vi "UnitTest-TimeLimitReliabilitycheck.vi"(8 "error in (no error)":errorcluster) -> (0 "error out":errorcluster)   [LabVIEW 2014]
uses:
  TableLogger_Actor/TableLoggerConfig.ctl
  TableLogger_Actor/TableLoggerTypes.ctl
  TableLogger_Actor/TableLoggerBackupConfig.ctl
  <vilib>/addons/_JKI Toolkits/Caraya/classes/Test/Test.lvclass
  TableLogger_Actor/TableLogger_Actor.lvlib
  <vilib>/addons/_JKI Toolkits/Caraya/classes/Assert/Assert.lvclass
panel:
  # "Connector Pane"
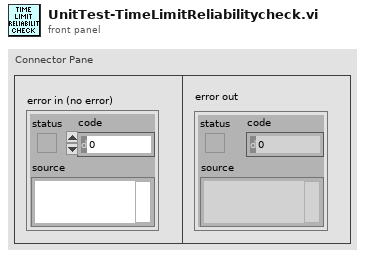
[diagram p1: front panel]
types:
  T1 = typedef "TableLogger_Actor.lvlib/TableLoggerConfig.ctl" = cluster{"TableLogger":T2, "DB File Path":path, "DB Backup Config":T3}
  T2 = typedef "TableLogger_Actor.lvlib/TableLoggerTypes.ctl" = enum16{"CSV Logger", "SQLite Logger"}
  T3 = typedef "TableLogger_Actor.lvlib/TableLoggerBackupConfig.ctl" = cluster{"Directory":path, "UTC Time Format":bool, "On Launch":bool, "Interval (Hours)":dbl, "Size Multiples (Bytes)":i32}
  T4 = typedef "TableLogger_Actor.lvlib/TableLoggerDataCluster.ctl" = cluster{"Numeric Data":i32, "Float Data":dbl, "String Data":string, "Enum Data":enum16{"Enum Item 1", "Enum Item 2"}, "Array Data":i32[]}
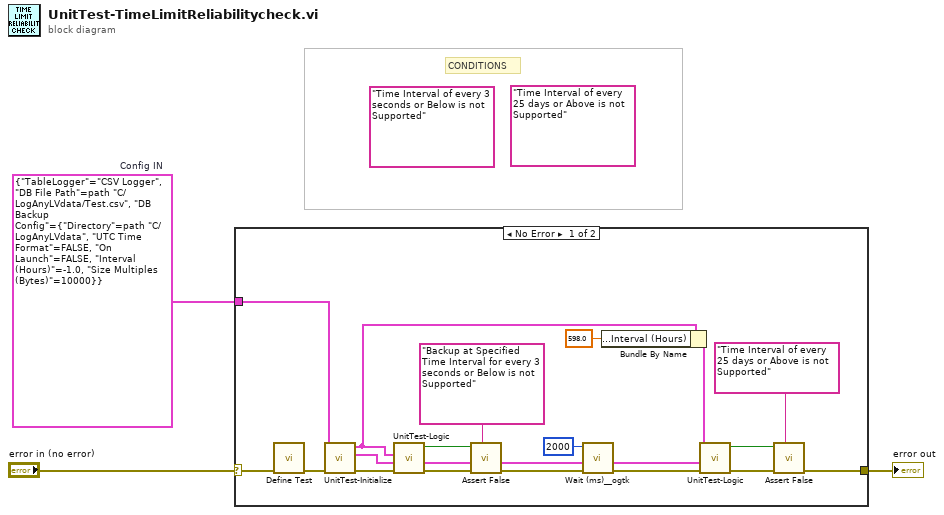
[diagram p0: block diagram]
diagram:
  w3 = T1 {"TableLogger"=enum."CSV Logger", "DB File Path"=path "C:/LogAnyLVdata/Test.csv", "DB Backup Config"={"Directory"=path "C:/LogAnyLVdata", "UTC Time Format"=FALSE, "On Launch"=FALSE, "Interval (Hours)"=-1.0, "Size Multiples (Bytes)"=10000}}  # Config IN
  (unwired) "Time Interval of every 25 days or Above is not Supported" ("Label")
  (unwired) "Time Interval of every 3 seconds or Below is not Supported" ("Label")
  # "CONDITIONS"
  n1 = case shown="No Error" "error in (no error)" {
    selector: "error in (no error)" -> [w21 w22]
    tunnel: [w14 w22] -> w1
    tunnel: w3 -> [w16 _]
    frame No Error {
      n2 = call <vilib>:"Define Test.vi"("error in (no error)"=w21) -> ("error out"=w20:errorcluster)  [unwired: 10 in]
      n3 = call "UnitTest-Initialize.vi"("error in"=w20, "Config IN"=w16) -> ("error out"=w19:errorcluster, "LV Data"=w9:T4, "Config OUT"=w10:T1)  [unwired: 7 in]
      n4 = call "UnitTest-Logic.vi"("error in (no error)"=w19, "LV Data"=w9, "TableLogger Config"=w10) -> ("error out"=w18:errorcluster, "Test Result"=w12:bool)  [unwired: 7 in]
      n5 = call <vilib>:"Assert False.vi"("Label"="Backup at Specified Time Interval for every 3 seconds or Below is not Supported", "error in (no error)"=w18, "False?"=w12) -> ("error out"=w17:errorcluster)  [unwired: 8 in]
      n6 = call "Wait (ms)__ogtk.vi"("error in (no error)"=w17, "milliseconds to wait"=u32 2000) -> ("error out"=w5:errorcluster)  [unwired: 8 in, 1 out]
      n7 = Bundle By Name(cluster=w10, "DB Backup Config.Interval (Hours)"=598.0) -> (w8:T1)
      n8 = call "UnitTest-Logic.vi"("error in (no error)"=w5, "LV Data"=w9, "TableLogger Config"=w8) -> ("error out"=w11:errorcluster, "Test Result"=w6:bool)  [unwired: 7 in]
      n9 = call <vilib>:"Assert False.vi"("Label"="Time Interval of every 25 days or Above is not Supported", "error in (no error)"=w11, "False?"=w6) -> ("error out"=w14:errorcluster)  [unwired: 8 in]
    }
    frame Error {
    }
  }
  "error out" <- w1
